vi "Play Editor.vi"() -> ()   [LabVIEW 2014]
uses:
  Autonomous VIs/Autonomous Exec/Autonomous Play Definition.ctl
  Autonomous VIs/Autonomous Commands/Autonomous Command Names.ctl
  <vilib>/FTP/NI_FTP.lvlib
panel:
  in  "Reload\nFolder":bool
  out "Error \nSending \nFiles":errorcluster
  out "Error \nRetrieving \nFiles":errorcluster
  in  "Empty Play Definition":T1 caption="Play"
  in  "Robot IP Address":string="10.xx.yy.2"
  in  "Download Plays":bool
  in  "Connected to Robot":bool
  in  "Send Plays":bool
  out "Create Play Error":errorcluster
  out "Play Read Error":errorcluster
  in  "Static Form":bool
  out "Commit Play Error":errorcluster
  in  "Current File Refnum":refnum<file>
  in  "Is a File":bool
  in  "Commit Play Changes":bool
  in  "Auto Directory":path
  in  "Finish":bool
  in  "Current Directory":path
  in  "Create New Play":bool
  in  "Play Currently Open":T1 caption="Play"
  in  "Play Selector Box":string(combo)
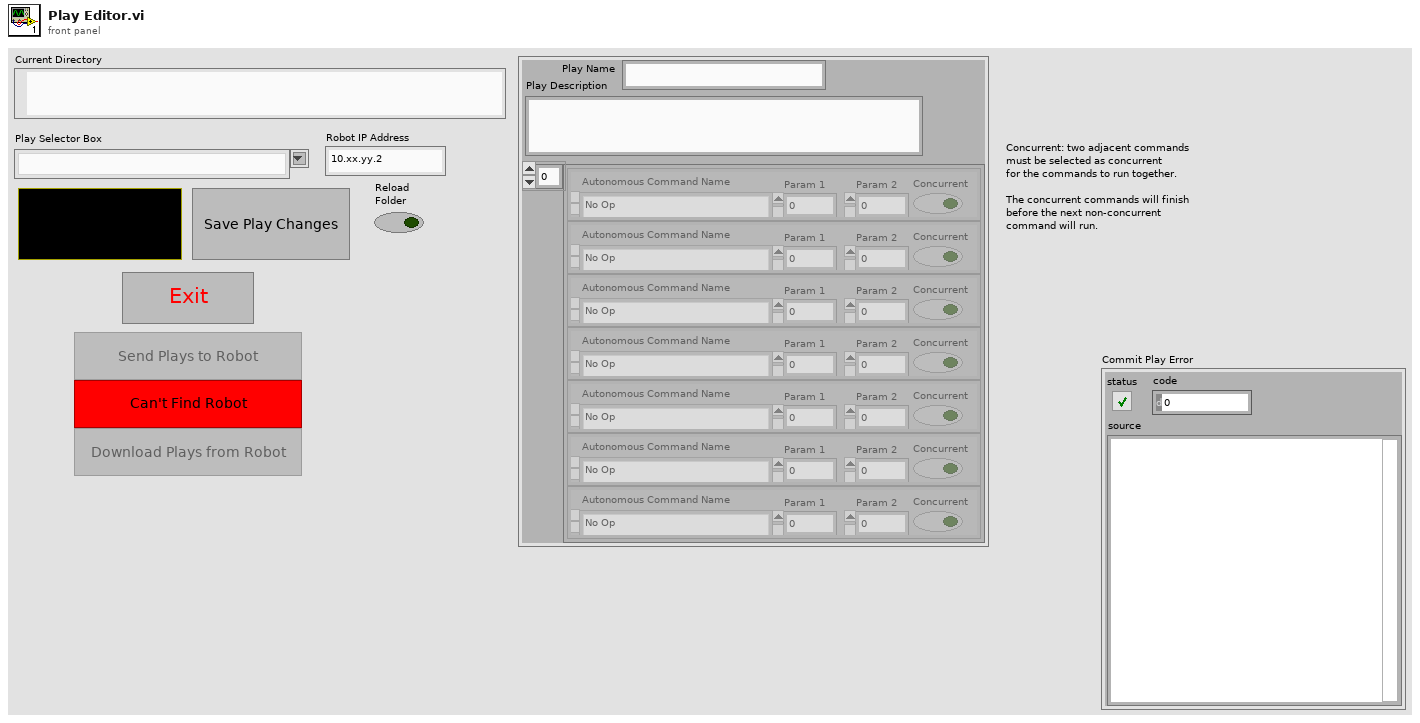
[diagram p1: front panel]
types:
  T1 = typedef "Autonomous Play Definition.ctl" = cluster{"Play Name":string, "Command List":cluster{"Param 1":dbl, "Param 2":dbl, "Autonomous Command Name":T2, "Concurrent":bool}[], "Play Description":string}
  T2 = typedef "Autonomous Command Names.ctl" = enum16{"No Op", "Drive Distance Robot", "Drive Time Robot", "Translate Distance Robot", "Translate Time Robot", "Drive Distance Field", "Drive Time Field", "Translate Distance Field", "Translate Time Field", "Rotate Robot", "Set Initial Gyro Value", "Lifter to Setpoint", "Wait", "Do Not use", "Drive Distance Field (Gyro Hold)", "Translate Distance Field (Gyro Hold)", "Can", "Grabber", "Drive Distance Field (Sensor Stop, Gyro Hold)", "Move Direction Field (Gyro Hold)", "Rotate Robot 90 about Tote", "Reset Gyro", "Find Tote", "Get Tote Into Robot", "Lower Can Grabber"}
  T3 = typedef "NI_FTP.lvlib/FTP Session.ctl" = refnum<k5>
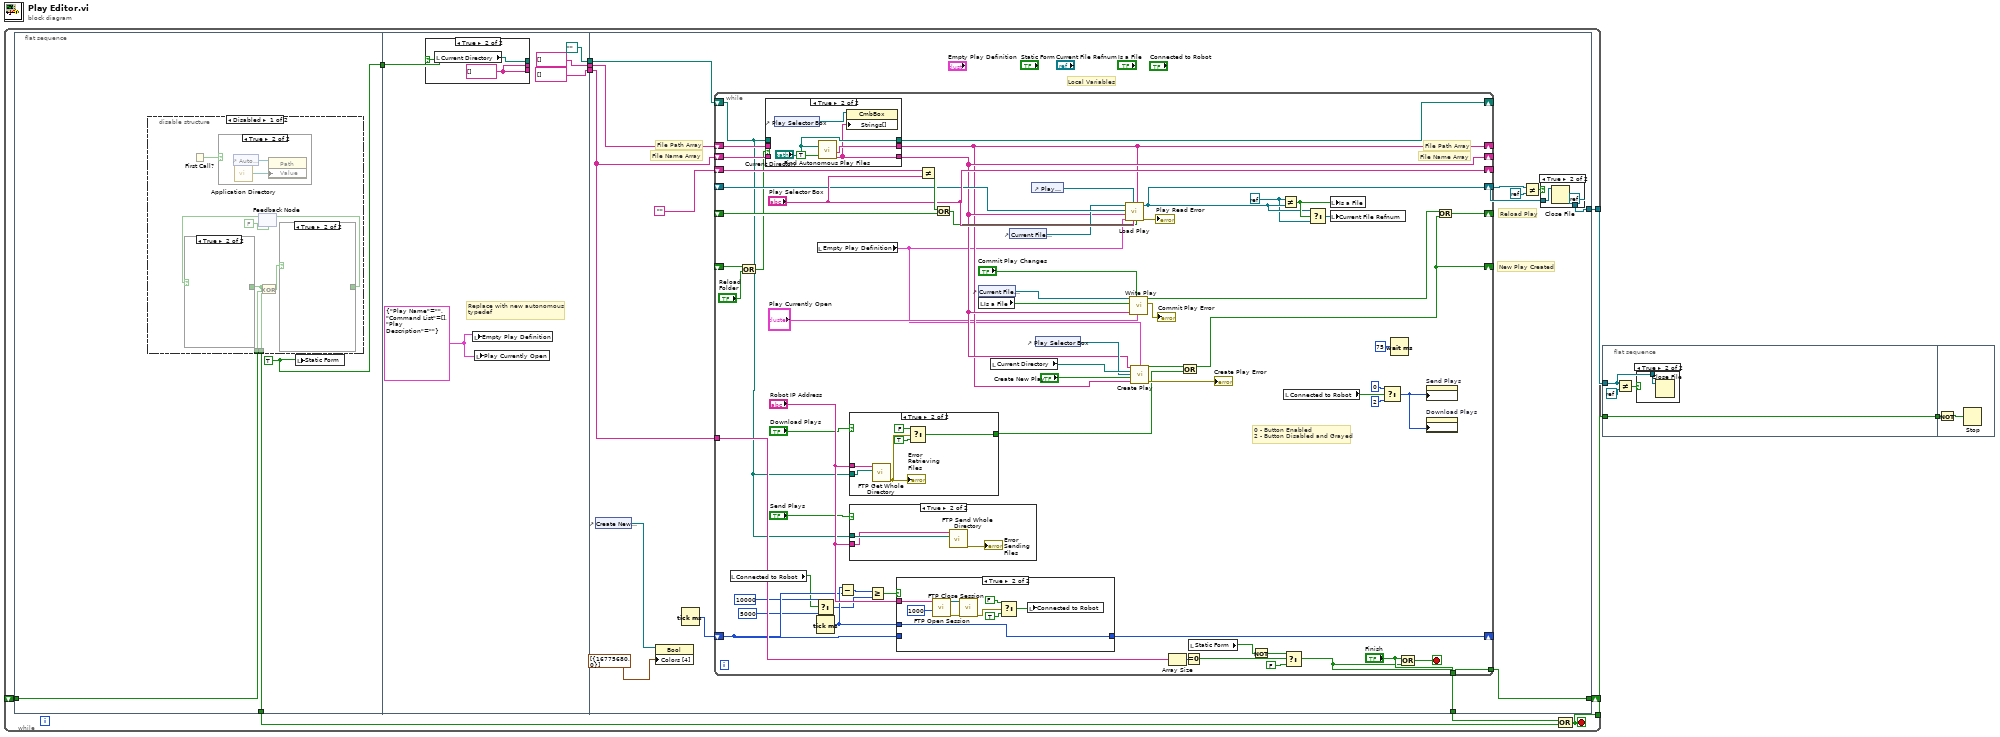
[diagram p0: block diagram]
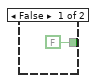
[diagram p3: hidden frame]
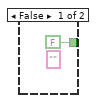
[diagram p4: hidden frame]
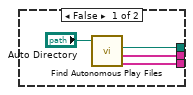
[diagram p7: hidden frame]
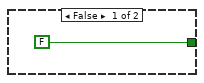
[diagram p11: hidden frame]
diagram:
  n1 = while {
    shift-right: [w10] -> _
    shift-left: _ -> [w9]
    tunnel: [w7] -> w2
    tunnel: [w6] -> w1
    stop <- w7 stop-if-true
    n2 = flat-sequence {
      tunnel: [w15] -> w8
      tunnel: w9 -> [w16]
      tunnel: [w14] -> w4
      tunnel: [string[] [] ("Filepath Array")] -> w13
      tunnel: [path "" ("Current Directory")] -> w12
      tunnel: [string[] [] ("Filepath Array")] -> w5
      tunnel: w4 -> [w32]
      tunnel: w13 -> [w41]
      tunnel: w12 -> [w39]
      tunnel: [w48] -> w11
      tunnel: [w45] -> w10
      tunnel: [w42] -> w6
      tunnel: w5 -> [w43]
      frame #0 {
        w14 = TRUE ("Static Form")
        n3 = disable-structure shown="Disabled" {
          disable-tunnel: w16 -> [w22 _]
          disable-tunnel: [w17 _] -> w15
          frame Disabled {
            n4 = First Call?() -> (First Call?: T/F=w23:bool)
            n5 = case shown="True" w23 {
              frame False {
              }
              frame True {
                n6 = control-ref of="Auto Directory"() -> (w27:refnum<vi>)
                n7 = call <vilib>:"Application Directory.vi"() -> ("Application Directory"=w26:path)
                n8 = property class="Path"(reference=w27, "Value"=w26) -> ()  [unwired: 1 in, 2 out]
              }
            }
            n9 = feedback #1(FALSE ("OK")) -> (w19:bool)
            n10 = case shown="True" w19 {
              tunnel: [FALSE ("No") _] -> w17
              frame False {
              }
              frame True {
              }
            }
            n11 = Exclusive Or(1:w22, 2:w17) -> (0:w21:bool)
            n12 = case shown="True" w21 {
              tunnel: [FALSE ("OK") _] -> w20
              frame False {
                (unwired) "" ("Full Directory")
              }
              frame True {
              }
            }
            n13 = feedback-in #1(w20) -> ()
          }
          frame Enabled {
          }
        }
        n14 = local write "Static Form"(w14) -> ()
      }
      frame #1 {
        w31 = T1 {"Play Name"="", "Command List"=[], "Play Description"=""} ("Play 1")
        # "Replace with new autonomous\ntypedef"
        n15 = case shown="True" w32 {
          tunnel: [w35 w37] -> _
          tunnel: [w34 w38] -> _
          tunnel: [w33 w38] -> _
          frame False {
            n16 = call "Find Autonomous Play Files.vi"("Application Directory"="Auto Directory") -> ("Application Directory"=w35:path, "Filepath Array"=w33:string[], "filename array"=w34:string[])  [unwired: 2 in, 1 out]
          }
          frame True {
            w38 = string[] [] ("Filepath Array")
            n17 = local read "Current Directory"() -> (w37:path)
          }
        }
        n18 = local write "Empty Play Definition"(w31) -> ()
        n19 = local write "Play Currently Open"(w31) -> ()
      }
      frame #2 {
        # "Local Variables"
        # "File Path Array"
        # "File Name Array"
        # "New Play Created"
        # "Reload Play"
        n20 = control-ref of="Create New Play"() -> (w50:refnum<vi>)
        n21 = property class="Bool"(reference=w50, "Colors [4]"=cluster{u32, u32}[] [{16775680, 0}]) -> ()  [unwired: 1 in, 2 out]
        n22 = Tick Count (ms)() -> (millisecond timer value=w40:u32)
        n23 = while {
          shift-right: ["Play Selector Box"] -> _
          shift-left: "" -> [w117]
          shift-right: [w108] -> w44
          shift-left: _ -> [w114]
          shift-right: [w92] -> _
          shift-left: _ -> [w104]
          tunnel: w41 -> [w112]
          tunnel: ["Finish"] -> w48
          tunnel: [w97] -> w45
          shift-right: [w61] -> _
          shift-left: _ -> [w58]
          shift-right: [w82] -> _
          shift-left: w43 -> [w94]
          shift-right: [w83] -> _
          shift-left: w41 -> [w93]
          shift-right: [w75] -> _
          shift-left: w40 -> [w71]
          shift-right: [w56] -> _
          shift-left: w39 -> [w55]
          stop <- w113 stop-if-true
          w106 = refnum<k0> refnum
          # "0 - Button Enabled\n2 - Button Disabled and Grayed"
          # "File Path Array"
          # "File Name Array"
          n24 = local read "Connected to Robot"() -> (w64:bool)
          n25 = Or(x=w58, y="Reload\nFolder") -> (x .or. y?=w59:bool)
          n26 = case shown="True" w59 {
            tunnel: [w140 w145] -> w82
            tunnel: [w139 w141] -> w83
            tunnel: w94 -> [w140 _]
            tunnel: w93 -> [w139 _]
            tunnel: w55 -> [w138 _]
            tunnel: [w138 "Current Directory"] -> w56
            frame False {
            }
            frame True {
              n27 = control-ref of="Play Selector Box"() -> (w142:refnum<vi>)
              n28 = call "Find Autonomous Play Files.vi"("Application Directory"="Current Directory", "Do not include file\nsuffix"=TRUE ("Do not include\nstring ending")) -> ("Filepath Array"=w145:string[], "filename array"=w141:string[])  [unwired: 1 in, 2 out]
              n29 = property class="CmbBox"(reference=w142, "Strings[]"=w141) -> ()  [unwired: 1 in, 2 out]
            }
          }
          n30 = Select(t=u32 10000 ("y"), s=w64, f=u32 5000 ("y")) -> (s? t:f=w69:u32)
          n31 = Tick Count (ms)() -> (millisecond timer value=w74:u32)
          n32 = local read "Empty Play Definition"() -> (w66:T1)
          n33 = Subtract(x=w74, y=w71) -> (x-y=w73:u32)
          n34 = case shown="True" "Download Plays" {
            tunnel: w55 -> [_ w137]
            tunnel: "Robot IP Address" -> [_ w136]
            tunnel: [FALSE ("Load New Play") w132] -> w60
            frame False {
            }
            frame True {
              n35 = call "FTP Get Whole Directory.vi"("Local Folder of Autonomous Plays"=w137, "host"=w136) -> ("error out"=w135:errorcluster)  [unwired: 9 in]
              "Error \nRetrieving \nFiles" <- w135
              n36 = Select(t=FALSE, s=w135, f=TRUE ("Load New Play")) -> (s? t:f=w132:bool)
            }
          }
          n37 = case shown="True" "Send Plays" {
            tunnel: w55 -> [_ w130]
            tunnel: "Robot IP Address" -> [_ w129]
            frame False {
            }
            frame True {
              n38 = call "FTP Send Whole Directory.vi"("Local Folder of Autonomous Plays"=w130, "host"=w129) -> ("error out"=→"Error \nSending \nFiles":errorcluster)  [unwired: 9 in]
            }
          }
          n39 = Greater Or Equal?(x=w73, y=w69) -> (x >= y?=w72:bool)
          n40 = case shown="True" w72 {
            tunnel: "Robot IP Address" -> [_ w127]
            tunnel: [w118 w119] -> w75
            tunnel: w74 -> [_ w119]
            tunnel: w71 -> [w118 _]
            frame False {
            }
            frame True {
              n41 = call <vilib>:"FTP Open Session.vi"("timeout ms (60000)"=1000, "address"=w127) -> ("error out"=w124:errorcluster, "ftp session"=w125:T3)  [unwired: 6 in, 2 out]
              n42 = call <vilib>:"FTP Close Session.vi"("error in (no error)"=w124, "ftp session"=w125) -> ("error out"=w123:errorcluster)  [unwired: 6 in, 3 out]
              n43 = Select(t=FALSE, s=w123, f=TRUE) -> (s? t:f=w120:bool)
              n44 = local write "Connected to Robot"(w120) -> ()
            }
          }
          n45 = Not Equal?(x=w117, y="Play Selector Box") -> (x != y?=w116:bool)
          n46 = Or(x=w116, y=w104) -> (x .or. y?=w100:bool)
          n47 = control-ref of="Current File Refnum"() -> (w87:refnum<vi>)
          n48 = local read "Is a File"() -> (w88:bool)
          n49 = local read "Current Directory"() -> (w86:path)
          n50 = control-ref of="Current File Refnum"() -> (w90:refnum<vi>)
          n51 = control-ref of="Play Currently Open"() -> (w65:refnum<vi>)
          n52 = control-ref of="Play Selector Box"() -> (w85:refnum<vi>)
          n53 = call "Load Play.vi"("Load Play"=w100, "Filepath Array"=w82, "Play Selector Box"="Play Selector Box", "Play Currently Open Property Reference"=w65, "Empty Play Definition"=w66, "filename array"=w83, "Previous Iteration \nFile Refnum"=w114, "Current File Refnum"=w90) -> ("Read file error"=→"Play Read Error":errorcluster, "Output File Refnum"=w108:refnum<file>)  [unwired: 2 in]
          n54 = call "Write Play.vi"("Current Selected Play"="Play Currently Open", "Commit Play Changes"="Commit Play Changes", "filename array"=w83, "Is a File"=w88, "File Refnum"=w87) -> ("File Write Error"=→"Commit Play Error":errorcluster, "Not Cancelled\nLoad File"=w105:bool)  [unwired: 5 in]
          n55 = call "Create Play.vi"("Filename Array in"=w83, "Empty Play Definition"=w66, "Application Directory"=w86, "Play Selection Box Property Reference"=w85, "Create New Play"="Create New Play", "Filepath Array in"=w82) -> ("Load New Play"=w91:bool, "error out"=→"Create Play Error":errorcluster)  [unwired: 6 in, 2 out]
          n56 = Array Size(array=w112) -> (size(s)=w111:i32)
          n57 = Or(x=w91, y=w60) -> (x .or. y?=w61:bool)
          n58 = Equal To 0?(x=w111) -> (x = 0?=w99:bool)
          n59 = local read "Static Form"() -> (w98:bool)
          n60 = Not(x=w98) -> (.not. x?=w96:bool)
          n61 = Not Equal?(x=w106, y=w108) -> (x != y?=w109:bool)
          n62 = local read "Connected to Robot"() -> (w78:bool)
          n63 = Select(t=w96, s=w99, f=FALSE) -> (s? t:f=w97:bool)
          n64 = Select(t=w108, s=w109, f=w106) -> (s? t:f=w107:refnum<file>)
          n65 = local write "Is a File"(w109) -> ()
          n66 = local write "Current File Refnum"(w107) -> ()
          n67 = Select(t=0, s=w78, f=2) -> (s? t:f=w76:i32)
          n68 = Wait (ms)(milliseconds to wait=u32 75) -> ()  [unwired: 1 out]
          n69 = Compound Arithmetic op=OR("Finish", w97) -> (w113:bool)
          n70 = property on="Send Plays" class="Bool"("DisabledEnum"=w76) -> ()  [unwired: 2 in, 2 out]
          n71 = property on="Download Plays" class="Bool"("DisabledEnum"=w76) -> ()  [unwired: 2 in, 2 out]
          n72 = Or(x=w105, y=w61) -> (x .or. y?=w92:bool)
        }
        n73 = Not Equal?(x=w44, y=refnum<k0> refnum) -> (x != y?=w46:bool)
        n74 = case shown="True" w46 {
          tunnel: w44 -> [w52 w54]
          tunnel: [w52 refnum<k0> refnum] -> w42
          frame False {
          }
          frame True {
            n75 = Close File(refnum=w54) -> ()  [unwired: 1 in, 2 out]
          }
        }
      }
    }
    n76 = Compound Arithmetic op=OR(w11, w8) -> (w7:bool)
  }
  n77 = flat-sequence {
    tunnel: [w149] -> w3
    tunnel: w2 -> [w149]
    tunnel: w1 -> [w146]
    tunnel: w3 -> [w152]
    frame #0 {
      n78 = Not Equal?(x=w146, y=refnum<k0> refnum) -> (x != y?=w147:bool)
      n79 = case shown="True" w147 {
        tunnel: w146 -> [_ w150]
        frame False {
        }
        frame True {
          n80 = Close File(refnum=w150) -> ()  [unwired: 1 in, 2 out]
        }
      }
    }
    frame #1 {
      n81 = Not(x=w152) -> (.not. x?=w151:bool)
      n82 = Stop(stop? (T)=w151) -> ()
    }
  }
